vi "SetMenuActive.vi"(8 "error in (no error)":errorcluster, 10 "Active?":bool, 11 "Game in":refnum<class "Game.lvclass">) -> (0 "error out":errorcluster, 3 "Game out":refnum<class "Game.lvclass">)   [LabVIEW 2019, in "RT_Game.lvlib" / "Game.lvclass"]
uses:
  Game.lvclass
  Game.lvclass/Game.ctl
  GameMenu/GameMenu.lvclass/GameMenu.ctl
  GameMenu/Write Active_.vi
  GameMenu/GameMenu.lvclass
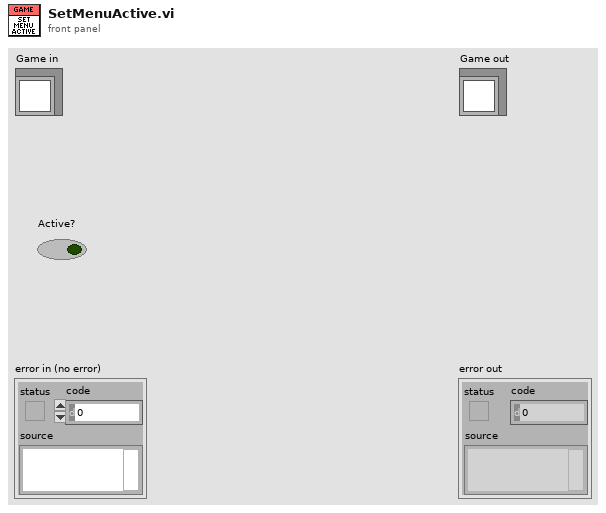
[diagram p1: front panel]
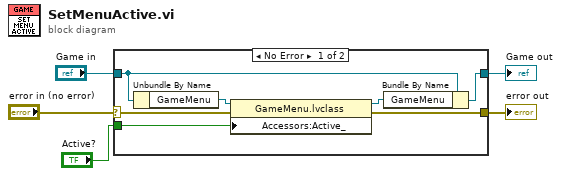
[diagram p0: block diagram]
diagram:
  n1 = case shown="No Error" "error in (no error)" {
    selector: "error in (no error)" -> [w12 w14]
    tunnel: [w9 w14] -> w4
    tunnel: [w10 w13] -> w2
    tunnel: "Game in" -> [w11 w13]
    tunnel: "Active?" -> [w6 _]
    frame No Error {
      n2 = Unbundle By Name(w11) -> ("GameMenu"=w8:refnum<class "GameMenu.lvclass">)
      n3 = property class="GameMenu.lvclass"(reference=w8, error in=w12, "Accessors:Active_"=w6) -> (reference out=w7:refnum<class "GameMenu.lvclass">, error out=w9:errorcluster)
      n4 = Bundle By Name(cluster=w11, "GameMenu"=w7) -> (w10:refnum<class "Game.lvclass">)
    }
    frame Error {
    }
  }
  "error out" <- w4
  "Game out" <- w2
